vi "Scale_in_range.vi"(7 "Scale Factor":dbl=1.0, 8 "Maximum Range":dbl=100.0, 9 "Minimum Range":dbl=-100.0, 11 "x":dbl) -> (3 "Scaled x":dbl)   [LabVIEW 2011]
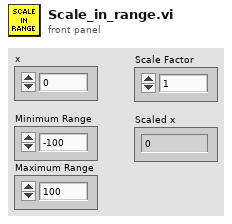
[diagram p1: front panel]
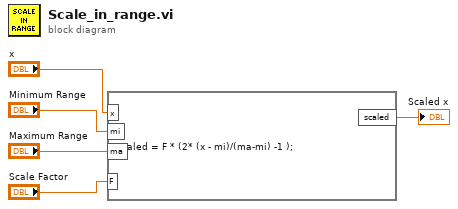
[diagram p0: block diagram]
diagram:
  n1 = formula code="scaled = F * (2* (x - mi)/(ma-mi) -1 );"("x"="x", "mi"="Minimum Range", "ma"="Maximum Range", "F"="Scale Factor") -> ("scaled"=→"Scaled x":dbl)
